vi "Write activeChannel.vi"(8 "error in (no error)":errorcluster, 10 "active axis":T1, 11 "HexapodPI in":refnum<class "HexapodPI.lvclass">) -> (0 "error out":errorcluster, 3 "HexapodPI out":refnum<class "HexapodPI.lvclass">)   [LabVIEW 2020, in "HexapodPI.lvclass"]
uses:
  HexapodPI.lvclass
  activeChannel.ctl
  HexapodPI.lvclass/HexapodPI.ctl
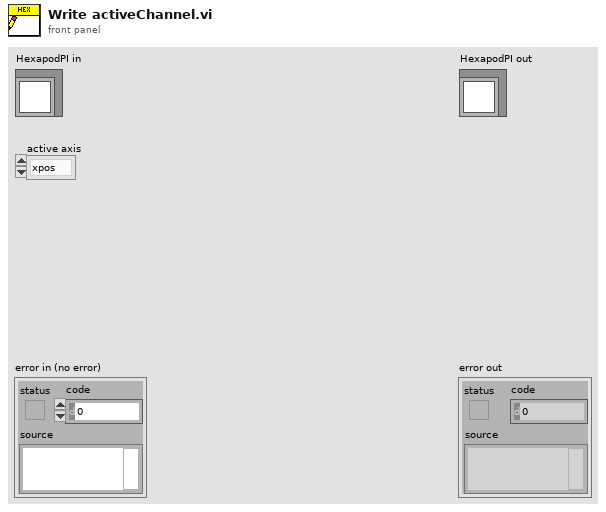
[diagram p1: front panel]
types:
  T1 = typedef "activeChannel.ctl" = enum16{"xpos", "ypos", "zpos", "uangle", "vangle", "wangle", "n/a", "off"}
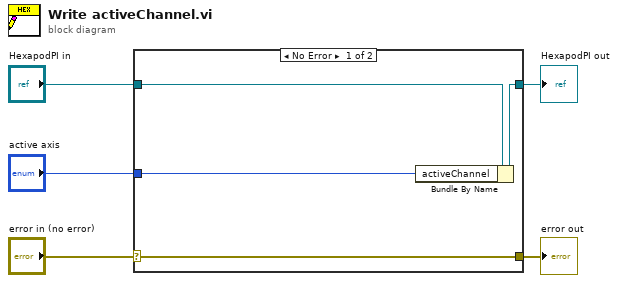
[diagram p0: block diagram]
diagram:
  n1 = case shown="No Error" "error in (no error)" {
    selector: "error in (no error)" -> [w9 w10]
    tunnel: [w9 w10] -> w4
    tunnel: [w7 w11] -> w2
    tunnel: "HexapodPI in" -> [w8 w11]
    tunnel: "active axis" -> [w6 _]
    frame No Error {
      n2 = Bundle By Name(cluster=w8, "activeChannel"=w6) -> (w7:refnum<class "HexapodPI.lvclass">)
    }
    frame Error {
    }
  }
  "error out" <- w4
  "HexapodPI out" <- w2
